vi "G#Debugger_PopulateActiveDebugTree.vi"(0 "Front Panel":refnum<vi>, 1 "Tree":refnum<vi>, 2 "Active Project":refnum<vi>, 5 "error in (no error)":errorcluster) -> (19 "error out":errorcluster)   [LabVIEW 2017, in "G#Debugger.lvlib"]
uses:
  <vilib>/addons/_AddQ/G#Debugger/G#Debugger.lvlib
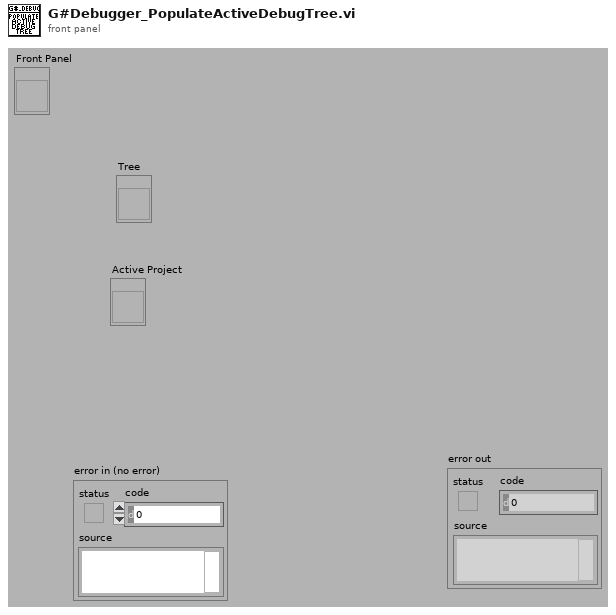
[diagram p1: front panel]
types:
  T1 = cluster{"Left Cell String":string, "Child Text":string[], "Child Tag":string, "Item Indent":i32, "Child Only?":bool, "Glyph Index":i32}
  T2 = cluster{"Left Cell String":string, "Child Text":string[], "Child Tag":string, "Item Indent":i32, "Child Only?":bool, "Glyph Index":i32}[]
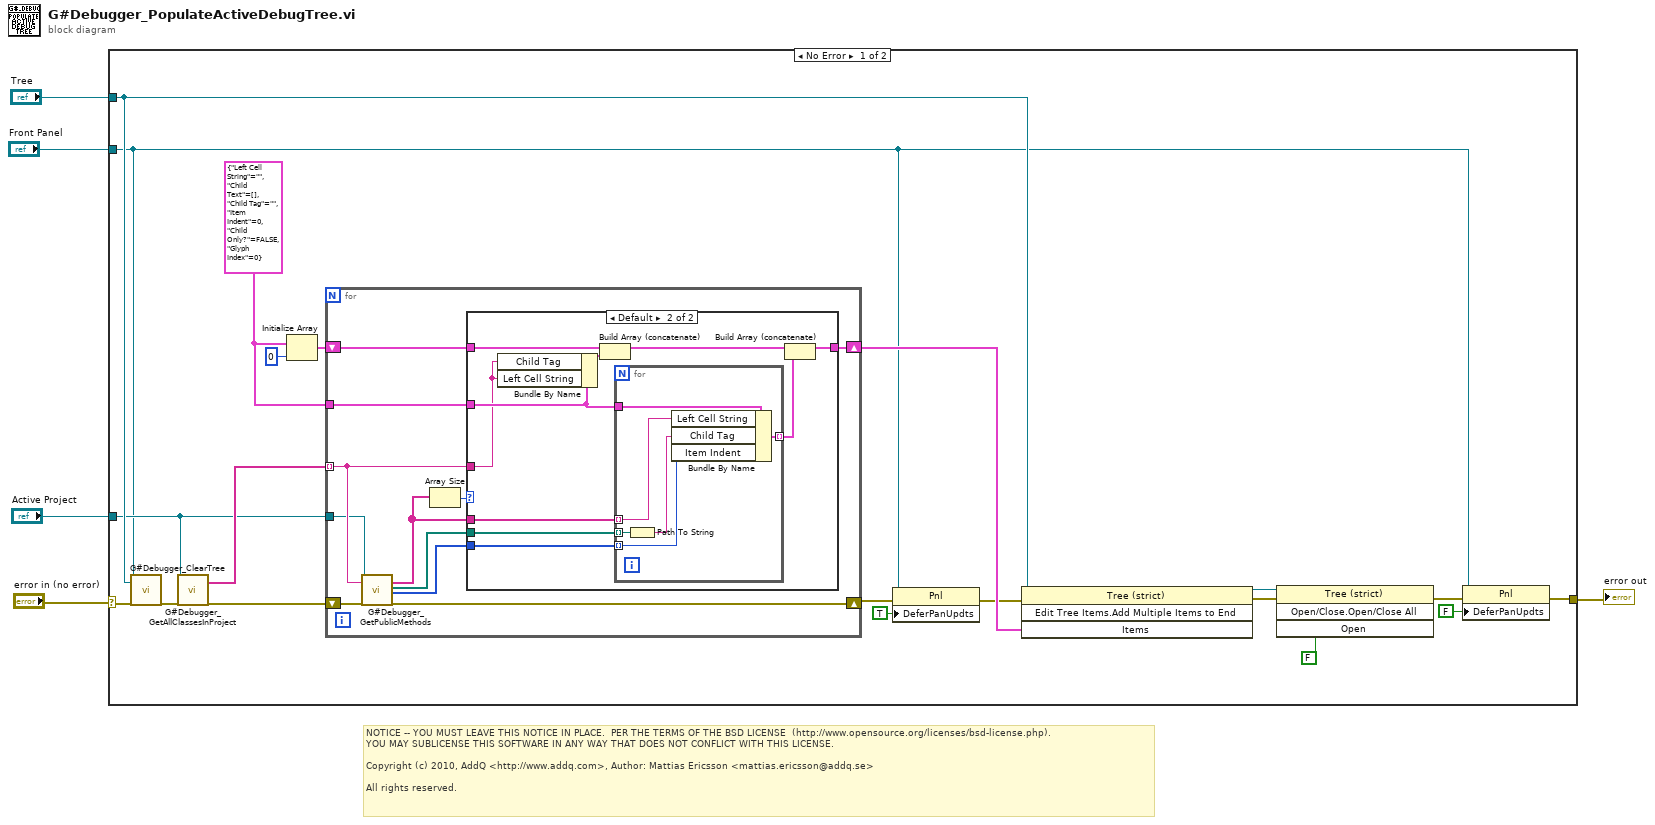
[diagram p0: block diagram]
diagram:
  # "NOTICE -- YOU MUST LEAVE THIS NOTICE IN PLACE.  PER THE TERMS OF THE BSD LICENSE  (http://www.opensource.org/licenses/bsd-license.php).\nYOU MAY SUBLICENSE THIS SOFTWARE IN ANY WAY THAT DOES NOT CONFLICT WITH THIS LICENSE.\n\nCopyright (c) 2010, AddQ <http://www.addq.com>, Author: Mattias Ericsson <mattias.ericsson@addq.se>\n\nAll rights reserved."
  n1 = case shown="No Error" "error in (no error)" {
    selector: "error in (no error)" -> [w25 w54]
    tunnel: [w7 w54] -> w4
    tunnel: "Tree" -> [w21 _]
    tunnel: "Active Project" -> [w13 _]
    tunnel: "Front Panel" -> [w8 _]
    frame No Error {
      w20 = T1 {"Left Cell String"="", "Child Text"=[], "Child Tag"="", "Item Indent"=0, "Child Only?"=FALSE, "Glyph Index"=0} ("Item")
      n2 = call <vilib>:"G#Debugger_ClearTree.vi"("Front Panel"=w8, "Tree"=w21, "error in (no error)"=w25) -> ("error out"=w19:errorcluster)  [unwired: 16 in]
      n3 = call <vilib>:"G#Debugger_GetAllClassesInProject.vi"("Active Project"=w13, "error in (no error)"=w19) -> ("G#Classes"=w18:string[], "error out"=w17:errorcluster)  [unwired: 16 in]
      n4 = Initialize Array(w20, 0 ("dimension size")) -> (w24:T2)
      n5 = for {
        shift-right: [w34] -> w22
        shift-left: w24 -> [w36]
        tunnel: w20 -> [w35]
        tunnel: w18 -> [w32] mode=indexing
        shift-right: [w31] -> w12
        shift-left: w17 -> [w33]
        tunnel: w13 -> [w26]
        n6 = call <vilib>:"G#Debugger_GetPublicMethods.vi"("Active Project"=w26, "ClassName"=w32, "error in (no error)"=w33) -> ("Methods"=w29:string[], "MethodPaths"=w28:path[], "Item indent"=w27:i32[], "error out"=w31:errorcluster)  [unwired: 13 in]
        n7 = Array Size(array=w29) -> (size(s)=w30:i32)
        n8 = case shown="Default" w30 {
          tunnel: w36 -> [w37 w47]
          tunnel: w35 -> [_ w45]
          tunnel: [w37 w44] -> w34
          tunnel: w29 -> [_ w41]
          tunnel: w32 -> [_ w40]
          tunnel: w28 -> [_ w39]
          tunnel: w27 -> [_ w38]
          frame 0 {
            # "If no objects of the class, don't show!"
          }
          frame Default {
            n9 = Bundle By Name(cluster=w45, "Child Tag"=w40, "Left Cell String"=w40) -> (w46:T1)
            n10 = Build Array (concatenate)(w47, w46) -> (w42:T2)
            n11 = for {
              tunnel: w41 -> [w51] mode=indexing
              tunnel: w45 -> [w53]
              tunnel: [w52] -> w43 mode=indexing
              tunnel: w39 -> [w50] mode=indexing
              tunnel: w38 -> [w48] mode=indexing
              n12 = Path To String(path=w50) -> (string=w49:string)
              n13 = Bundle By Name(cluster=w53, "Left Cell String"=w51, "Child Tag"=w49, "Item Indent"=w48) -> (w52:T1)
            }
            n14 = Build Array (concatenate)(w42, w43) -> (w44:T2)
          }
        }
      }
      n15 = property class="Pnl"(reference=w8, error in=w12, "DeferPanUpdts"=TRUE ("Defer Panel Updates")) -> (error out=w11:errorcluster)  [unwired: 1 out]
      n16 = invoke class="Tree (strict)" method="Edit Tree Items.Add Multiple Items to End"(reference=w21, error in=w11, "Items"=w22) -> (reference out=w16:refnum<vi>, error out=w15:errorcluster)  [unwired: 1 in, 2 out]
      n17 = invoke class="Tree (strict)" method="Open/Close.Open/Close All"(reference=w16, error in=w15, "Open"=FALSE ("Open?")) -> (error out=w9:errorcluster)  [unwired: 1 in, 3 out]
      n18 = property class="Pnl"(reference=w8, error in=w9, "DeferPanUpdts"=FALSE ("Defer Panel Updates")) -> (error out=w7:errorcluster)  [unwired: 1 out]
    }
    frame Error {
    }
  }
  "error out" <- w4
